vi "ConvertCellToPosition.vi"(11 "cell name":string) -> (2 "position":cluster{"row":i32, "column":i32}, 3 "MS Office Parameter":T1)   [LabVIEW 2018]
uses:
  <vilib>/addons/_office/NI_ReportGenerationToolkit.lvlib
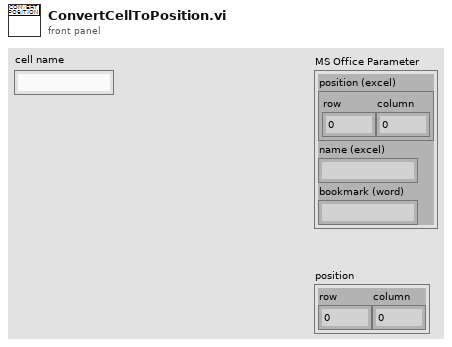
[diagram p1: front panel]
types:
  T1 = cluster{"position (excel)":cluster{"row":i32, "column":i32}, "name (excel)":string, "bookmark (word)":string}
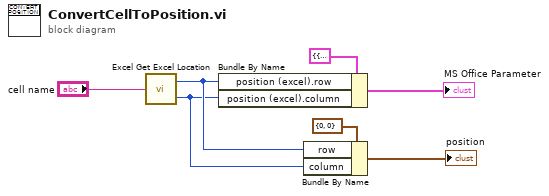
[diagram p0: block diagram]
diagram:
  n1 = call <vilib>:"Excel Get Excel Location.vi"("cell's name"="cell name") -> ("row"=w2:i32, "column"=w1:i32)
  n2 = Bundle By Name(cluster=T1 {"position (excel)"={"row"=0, "column"=0}, "name (excel)"="", "bookmark (word)"=""} ("MS Office parameters"), "position (excel).row"=w2, "position (excel).column"=w1) -> (→"MS Office Parameter":T1)
  n3 = Bundle By Name(cluster=cluster{"row":i32, "column":i32} {"row"=0, "column"=0} ("position"), "row"=w2, "column"=w1) -> (→"position":cluster{"row":i32, "column":i32})
